vi "Initialise.vi"(8 "error in (no error)":errorcluster, 10 "Message in":refnum<class "InitialiseMessage.lvclass">, 11 "Cascade in":refnum<class "Cascade.lvclass">) -> (0 "error out":errorcluster, 3 "Cascade out":refnum<class "Cascade.lvclass">)   [LabVIEW 2012, in "Cascade.lvclass"]
doc: "This method is called when an initialise message is received. It mainly initialises the RabbitMQ connectivity. \n\nOverride this method when your component needs special initialisation (e.g. of software or hardware resources). In that case, don't forget to call the parent for proper implementation. If your component owns subcomponents, they count as resources, so you have to initialise them by calling their own initialise functions"
uses:
  Cascade.lvclass
  <vilib>/Distrio/Murmex/InitialiseMessage/InitialiseMessage.lvclass
  <vilib>/Distrio/Murmex/Murmex/Murmex.lvclass
  data type.ctl
  Cascade.lvclass/Cascade.ctl
panel:
  # "This method is called when the INTIALISE\ntrigger is sent. \n\nOverride this method when your component needs to\nrespond to this trigger. \n\nCall parent for proper implementation"
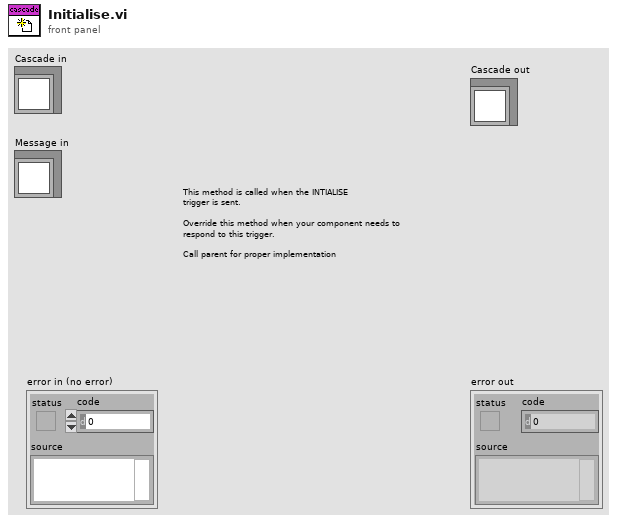
[diagram p1: front panel]
types:
  T1 = typedef "Image Type" = u32
  T2 = typedef "Cascade.lvclass/data type.ctl" = u32
  T3 = typedef "IMAQ Image.ctl" = refnum<image>
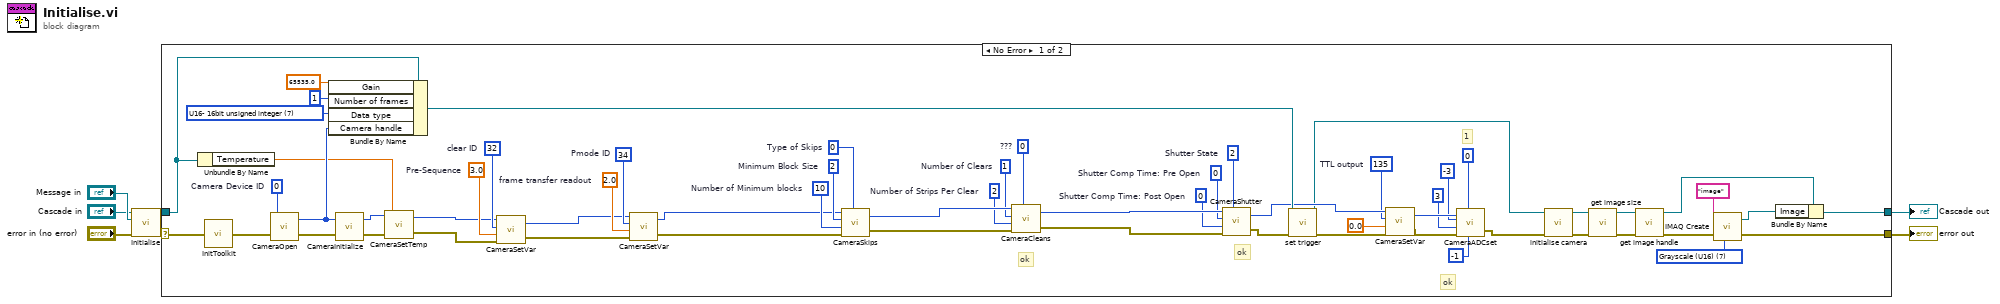
[diagram p0: block diagram]
diagram:
  n1 = call-parent "Initialise.vi"("error in (no error)"="error in (no error)", "Message in"="Message in", "Murmex in"="Cascade in") -> ("error out"=w4:errorcluster, "Murmex out"=w3:refnum<class "Cascade.lvclass">)  [unwired: 7 in]
  n2 = case shown="No Error" w4 {
    selector: w4 -> [w67 w69]
    tunnel: w3 -> [w39 w68]
    tunnel: [w46 w69] -> w2
    tunnel: [w45 w68] -> w1
    frame No Error {
      w25 = u32 135  # TTL output
      w37 = 2.0  # frame transfer readout
      w36 = u32 34  # Pmode ID
      w35 = 3.0  # Pre-Sequence
      w34 = u32 32  # clear ID
      w47 = T1 7 items=["Grayscale (U8)", "Grayscale (I16)", "Grayscale (SGL)", "Complex (CSG)", "RGB (U32)", "HSL (U32)", "RGB (U64)", "Grayscale (U16)"] ("Image Type")
      w49 = T2 7 items=["8bit signed integer"=1, "I16- 16bit signed integer"=2, "I32- 32bit signed integer"=3, "SGL- 32 bit floating point"=4, "DBL- 64 bit floating point"=5, "U8- 8bit unsigned"=6, "U16- 16bit unsigned integer"=7, "U32- 32 bit unsigned integer"=8] ("runtime.Data type")
      w52 = u32 0  # Shutter Comp Time: Post Open
      w53 = u32 0  # Shutter Comp Time: Pre Open
      w54 = u32 2  # Shutter State
      w55 = u32 2  # Number of Strips Per Clear
      w56 = u32 1  # Number of Clears
      w57 = u32 0  # ???
      w58 = u32 0  # Type of Skips
      w59 = u32 10  # Number of Minimum blocks
      w60 = u32 2  # Minimum Block Size
      w65 = u32 0  # Camera Device ID
      # "ok"
      # "ok"
      # "ok"
      # "1"
      n3 = Unbundle By Name(w39) -> ("Temperature"=w38:dbl)
      n4 = call <userlib>:"InitToolkit.vi"("error in"=w67) -> ("error out"=w66:errorcluster)
      n5 = call <userlib>:"CameraOpen.vi"("error in"=w66, "Camera Device ID"=w65) -> ("error out"=w43:errorcluster, "Camera Handle"=w42:u32)
      n6 = Bundle By Name(cluster=w39, "Gain"=65535.0 ("settings.Gain"), "Number of frames"=u32 1 ("settings.Number of frames"), "Data type"=w49, "Camera handle"=w42) -> (w50:refnum<class "Cascade.lvclass">)
      n7 = call <userlib>:"CameraInitialize.vi"("error in"=w43, "Camera Handle"=w42) -> ("error out"=w41:errorcluster, "Camera Handle"=w40:u32)
      n8 = call <userlib>:"CameraSetTemp.vi"("error in (no error)"=w41, "Temperature"=w38, "Camera Handle"=w40) -> ("error out"=w31:errorcluster, "Camera Handle"=w30:u32)
      n9 = call <userlib>:"CameraSetVar.vi"("error in"=w31, "Value"=w35, "Parameter ID"=w34, "Camera Handle"=w30) -> ("error out"=w32:errorcluster, "CameraHandle"=w33:u32)
      n10 = call <userlib>:"CameraSetVar.vi"("error in"=w32, "Value"=w37, "Parameter ID"=w36, "Camera Handle"=w33) -> ("error out"=w29:errorcluster, "CameraHandle"=w28:u32)
      n11 = call <userlib>:"CameraSkips.vi"("Camera Handle"=w28, "Minimum Block Size"=w60, "Number of Minimum blocks"=w59, "error in"=w29, "Type of Skips"=w58) -> ("Camera Handle"=w64:u32, "error out"=w63:errorcluster)
      n12 = call <userlib>:"CameraCleans.vi"("Camera Handle"=w64, "Number of Clears"=w56, "Number of Strips Per Clear"=w55, "error in"=w63, "Continuous Clears"=w57) -> ("Camera Handle"=w61:u32, "error out"=w62:errorcluster)
      n13 = call <userlib>:"CameraShutter.vi"("Camera Handle"=w61, "Shutter Comp Time: Pre Open"=w53, "Shutter Comp Time: Post Open"=w52, "error in"=w62, "Shutter State"=w54) -> ("Camera Handle"=w26:u32, "error out"=w51:errorcluster)
      n14 = call-dynamic "set trigger.vi"("error in (no error)"=w51, "Cascade in"=w50) -> ("error out"=w27:errorcluster, "Cascade out"=w9:refnum<class "Cascade.lvclass">)  [unwired: 8 in]
      n15 = call <userlib>:"CameraSetVar.vi"("error in"=w27, "Value"=0.0, "Parameter ID"=w25, "Camera Handle"=w26) -> ("error out"=w23:errorcluster, "CameraHandle"=w22:u32)
      n16 = call <userlib>:"CameraADCset.vi"("ADC offset"=-1, "Read Out port"=0, "error in (no error)"=w23, "ADC Gain"=3, "ADC Speed"=-3, "Camera Handle"=w22) -> ("error out"=w10:errorcluster)  [unwired: 1 out]
      n17 = call-dynamic "initialise camera.vi"("error in (no error)"=w10, "Cascade in"=w9) -> ("error out"=w18:errorcluster, "Cascade out"=w15:refnum<class "Cascade.lvclass">)  [unwired: 8 in]
      n18 = call-dynamic "get image size.vi"("error in (no error)"=w18, "Cascade in"=w15) -> ("error out"=w17:errorcluster, "Cascade out"=w14:refnum<class "Cascade.lvclass">)  [unwired: 8 in]
      n19 = call-dynamic "get image handle.vi"("error in (no error)"=w17, "Cascade in"=w14) -> ("error out"=w16:errorcluster, "Cascade out"=w13:refnum<class "Cascade.lvclass">)  [unwired: 8 in]
      n20 = call "IMAQ Create"("Image Name"="image", "Image Type"=w47, "error in (no error)"=w16) -> ("New Image"=w44:T3, "error out"=w46:errorcluster)  [unwired: 2 in]
      n21 = Bundle By Name(cluster=w13, "Image"=w44) -> (w45:refnum<class "Cascade.lvclass">)
    }
    frame Error {
    }
  }
  "error out" <- w2
  "Cascade out" <- w1
